vi "Test - Obtaining Unknown Object References Target.vi"() -> ()   [LabVIEW 2019]
doc: "This VI serves as the target VI for the Obtaining Unknown Object References.vi example. This VI intentionally does not show the labels of the controls and indicators on the block diagram so that the Obtaining Unknown Object References.vi example can use VI Scripting to programmatically display the labels of the controls and indicators in this VI.\n\nDo not save changes to this VI."
panel:
  out "Slide":dbl(slide) scale=0.0..10.0
  in  "Numeric 2":dbl
  in  "Numeric":dbl
  # "Select Help>>Show Context Help and move the cursor over the VI icon to display help for this VI.\n\nThis VI intentionally does not show the labels of the controls and indicators on the block diagram so that it can serve as the target VI for the Obtaining Unknown Object References.vi example, which uses VI Scripting to programmatically display the labels of the controls and indicators in this VI.\n\nDO NOT SAVE CHANGES TO THIS VI. Changing this VI might prevent the Obtaining Unknown Object References.vi example from demonstrating its scripting task."
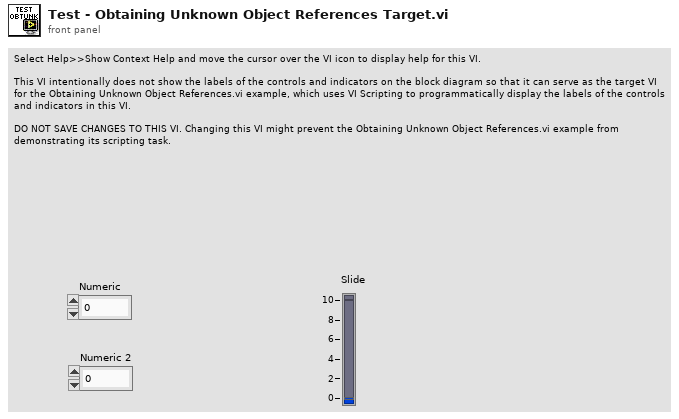
[diagram p1: front panel]
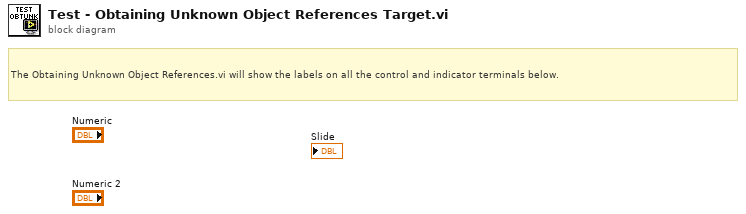
[diagram p0: block diagram]
diagram:
  # "The Obtaining Unknown Object References.vi will show the labels on all the control and indicator terminals below."
